vi "Test Sqrt Sqrt.vi"() -> ()   [LabVIEW 2014]
uses:
  <vilib>/Aledyne-TSXperts/Arduino Compatible Compiler for LabVIEW/addons/Complex Numbers/Complex Numbers.lvlib
panel:
  out "sqrt(A)":u32
  out "sqr(A)":u32
  out "Error Out":errorcluster
  in  "Error In":errorcluster
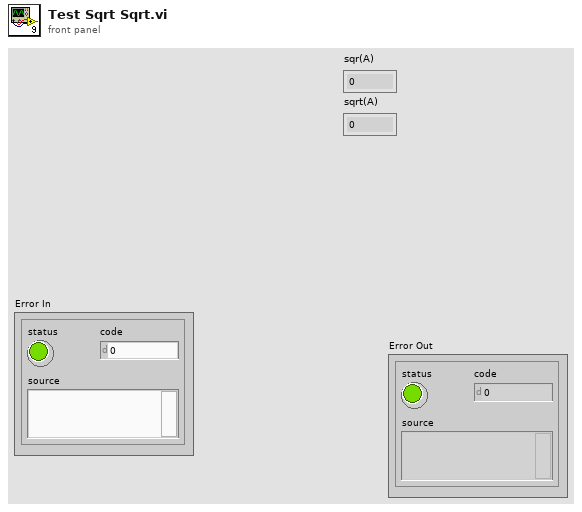
[diagram p1: front panel]
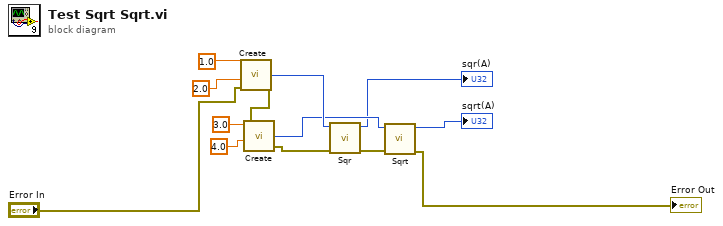
[diagram p0: block diagram]
diagram:
  n1 = call <vilib>:"Create.vi"("Error In"="Error In", "Imag"=2.0 ("Real"), "Real"=1.0) -> ("Error Out"=w10:errorcluster, "Complex"=w6:u32)  [unwired: 2 in]
  n2 = call <vilib>:"Create.vi"("Error In"=w10, "Imag"=4.0 ("Real"), "Real"=3.0) -> ("Error Out"=w7:errorcluster, "Complex"=w3:u32)  [unwired: 2 in]
  n3 = call <vilib>:"Sqr.vi"("Error In"=w7, "A"=w6) -> ("Error Out"=w5:errorcluster, "sqr(A)"=→"sqr(A)":u32)  [unwired: 8 in]
  n4 = call <vilib>:"Sqrt.vi"("Error In"=w5, "A"=w3) -> ("Error Out"=→"Error Out":errorcluster, "sqrt(A)"=→"sqrt(A)":u32)  [unwired: 8 in]
